vi "Set Return Variable (Boolean).vi"(8 "error in (no error)":errorcluster, 9 "Value":bool, 10 "Identifier":string, 11 "Sequence Ref in":refnum<k24>) -> (0 "error out":errorcluster, 3 "Sequence Ref out":refnum<k24>)   [LabVIEW 2015, in "Single Station Execution.lvlib"]
uses:
  Single Station Execution.lvlib
  NationalInstruments.VeriStand.RealTimeSequenceDefinitionApi
  NationalInstruments.VeriStand.DataTypes
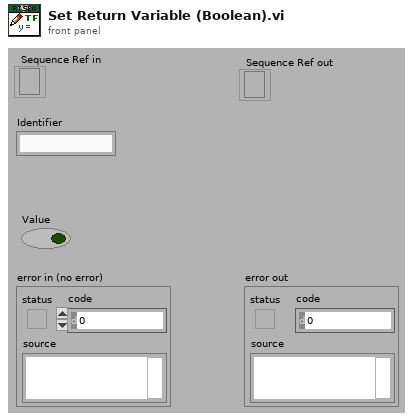
[diagram p1: front panel]
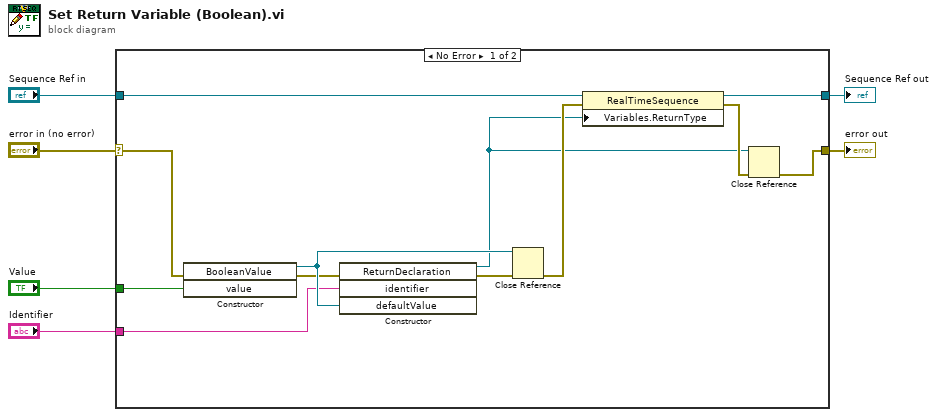
[diagram p0: block diagram]
diagram:
  n1 = case shown="No Error" "error in (no error)" {
    selector: "error in (no error)" -> [w9 w19]
    tunnel: "Value" -> [w15 _]
    tunnel: "Identifier" -> [w14 _]
    tunnel: "Sequence Ref in" -> [w13 w20]
    tunnel: [w12 w20] -> w3
    tunnel: [w10 w19] -> w2
    frame No Error {
      n2 = constructor class="BooleanValue"(error in=w9, "value"=w15) -> (reference out=w17:refnum<k24>, error out=w16:errorcluster)  [unwired: 2 in, 2 out]
      n3 = constructor class="ReturnDeclaration"(error in=w16, "identifier"=w14, "defaultValue"=w17) -> (reference out=w7:refnum<k24>, error out=w11:errorcluster)  [unwired: 2 in, 3 out]
      n4 = Close Reference(reference=w17, error in (no error)=w11) -> (error out=w18:errorcluster)
      n5 = property class="RealTimeSequence"(reference=w13, error in=w18, "Variables.ReturnType"=w7) -> (reference out=w12:refnum<k24>, error out=w8:errorcluster)
      n6 = Close Reference(reference=w7, error in (no error)=w8) -> (error out=w10:errorcluster)
    }
    frame Error {
    }
  }
  "Sequence Ref out" <- w3
  "error out" <- w2
